vi "Create Object.vi"(8 "error in (no error)":errorcluster, 10 "Object Name":string, 11 "CS++Factory in":refnum<class "CS++Factory.lvclass">) -> (0 "error out":errorcluster, 3 "CS++Factory out":refnum<class "CS++Factory.lvclass">)   [LabVIEW 2012, in "CS++BaseClasses.lvlib" / "CS++Factory.lvclass"]
doc: "Create an object by name. Object name is a kind of reference to attribute initialization data."
uses:
  CS++Factory.lvclass
  Base/CS++Base.lvclass
  Actors/CS++BaseActor/CS++BaseActor.lvclass
panel:
  out "Found?":bool
  out "LabVIEW Object":refnum<class>
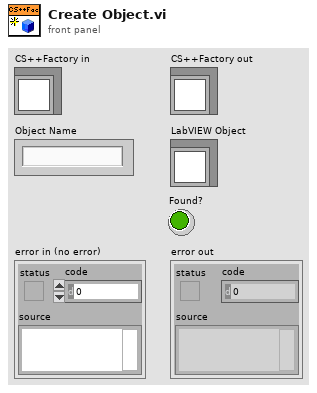
[diagram p1: front panel]
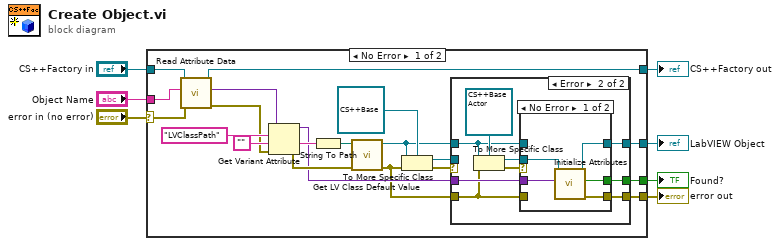
[diagram p0: block diagram]
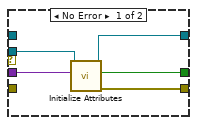
[diagram p2: hidden frame]
diagram:
  n1 = case shown="No Error" "error in (no error)" {
    selector: "error in (no error)" -> [w12 w50]
    tunnel: [w13 w50] -> w6
    tunnel: [w26 w49] -> w4
    tunnel: "CS++Factory in" -> [w27 w49]
    tunnel: [w14 _] -> w3
    tunnel: "Object Name" -> [w25 _]
    tunnel: [w11 _] -> w1
    frame No Error {
      n2 = call-dynamic "Read Attribute Data.vi"("error in (no error)"=w12, "Object Name"=w25, "CS++Factory in"=w27) -> ("error out"=w21:errorcluster, "Attribute Data"=w24:variant, "CS++Factory out"=w26:refnum<class "CS++Factory.lvclass">)  [unwired: 6 in]
      n3 = Get Variant Attribute(Variant=w24, name="LVClassPath", default value (empty Variant)="", error in=w21) -> (duplicate Variant=w15:variant, value=w20:string, error out=w18:errorcluster)  [unwired: 1 out]
      n4 = String To Path(string=w20) -> (path=w19:path)
      n5 = call <vilib>:"Get LV Class Default Value.vi"("error in (no error)"=w18, "class path"=w19) -> ("error out"=w8:errorcluster, "object"=w9:refnum<class>)  [unwired: 8 in]
      n6 = To More Specific Class(target class=refnum<class "CS++Base.lvclass"> refnum ("CS++BaseClasses.lvlib:CS++Base.lvclass"), reference=w9, error in=w8) -> (specific class reference=w16:refnum<class "CS++Base.lvclass">, error out=w10:errorcluster)
      n7 = case shown="Error" w10 {
        tunnel: w16 -> [w32 _]
        tunnel: w15 -> [w31 w36]
        tunnel: [w30 w38] -> w14
        tunnel: [w29 w35] -> w13
        tunnel: [w28 w34] -> w11
        tunnel: w9 -> [_ w37]
        tunnel: w8 -> [_ w33]
        frame No Error {
          n8 = call-dynamic "Initialize Attributes.vi"("Attribute Data"=w31, "CS++Base in"=w32) -> ("error out"=w29:errorcluster, "Found?"=w28:bool, "CS++Base out"=w30:refnum<class "CS++Base.lvclass">)  [unwired: 7 in]
        }
        frame Error {
          n9 = To More Specific Class(target class=refnum<class "CS++BaseActor.lvclass"> refnum ("CS++BaseActor.lvlib:CS++BaseActor.lvclass"), reference=w37, error in=w33) -> (specific class reference=w40:refnum<class "CS++BaseActor.lvclass">, error out=w39:errorcluster)
          n10 = case shown="No Error" w39 {
            tunnel: w40 -> [w46 _]
            tunnel: [w45 w48] -> w38
            tunnel: w37 -> [_ w48]
            tunnel: w36 -> [w44 _]
            tunnel: [w43 w47] -> w35
            tunnel: [w42 _] -> w34
            tunnel: w33 -> [_ w47]
            frame No Error {
              n11 = call-dynamic "Initialize Attributes.vi"("Attribute Data"=w44, "CS++BaseActor in"=w46) -> ("error out"=w43:errorcluster, "Found?"=w42:bool, "CS++BaseActor out"=w45:refnum<class "CS++BaseActor.lvclass">)  [unwired: 7 in]
            }
            frame Error {
            }
          }
        }
      }
    }
    frame Error {
    }
  }
  "error out" <- w6
  "CS++Factory out" <- w4
  "LabVIEW Object" <- w3
  "Found?" <- w1
